vi "实验2_2全局.vi"() -> ()   [LabVIEW 2018]
panel:
  in  "stop":bool
  in  "Numeric":dbl
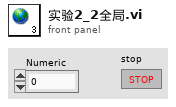
[diagram p1: front panel]
diagram:
